vi "EvaluatePoint.vi"(8 "error in (no error)":errorcluster, 9 "Game":refnum<class "Game.lvclass">, 10 "Point":dbl[](array[numeric]), 11 "SecondLevelThreat in":refnum<class "SecondLevelThreat.lvclass">) -> (0 "error out":errorcluster, 2 "Evaluation":dbl, 3 "SecondLevelThreat out":refnum<class "SecondLevelThreat.lvclass">)   [LabVIEW 2023, in "SecondLevelThreat.lvclass"]
uses:
  SecondLevelThreat.lvclass
  Game_class/Game.lvclass
  Evaluator_class/Evaluator.lvclass
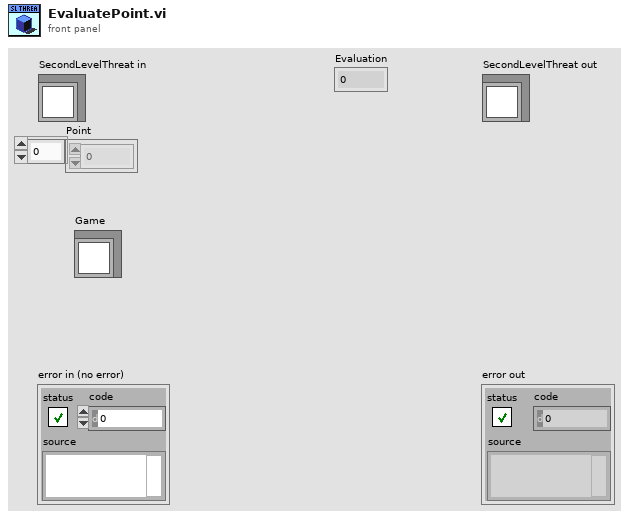
[diagram p1: front panel]
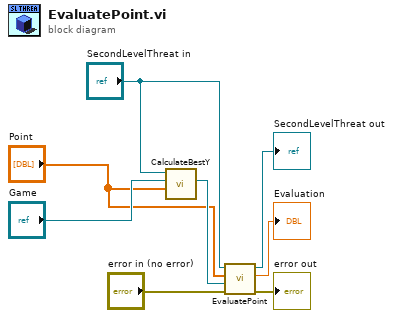
[diagram p0: block diagram]
diagram:
  n1 = call-dynamic "CalculateBestY.vi"("Point"="Point", "Game"="Game", "Evaluator in"="SecondLevelThreat in") -> ("Game out"=w2:refnum<class "Game.lvclass">)  [unwired: 6 in, 2 out]
  n2 = call-parent "EvaluatePoint.vi"("error in (no error)"="error in (no error)", "Game"=w2, "Point"="Point", "Evaluator in"="SecondLevelThreat in") -> ("error out"=→"error out":errorcluster, "Evaluation"=→"Evaluation":dbl, "Evaluator out"=→"SecondLevelThreat out":refnum<class "SecondLevelThreat.lvclass">)  [unwired: 5 in]
